vi "PWM.vi"(11 "Knob":dbl(knob) scale=0.0..100.0) -> (3 "s? t:f":bool)   [LabVIEW 2016]
panel:
  out "Waveform Chart":i16(graph)
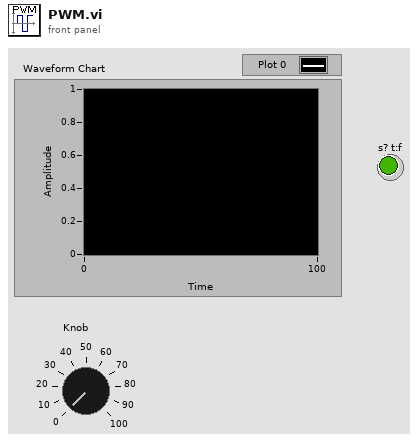
[diagram p1: front panel]
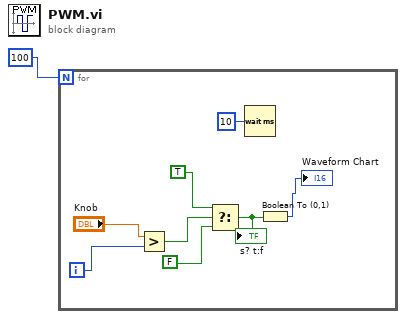
[diagram p0: block diagram]
diagram:
  n1 = for {
    N: 100 -> [_]
    i -> [w9]
    n2 = Greater?(x="Knob", y=w9) -> (0:w8:bool)
    n3 = Select(t=TRUE, s=w8, f=FALSE) -> (s? t:f=w4:bool)
    "s? t:f" <- w4
    n4 = Wait (ms)(milliseconds to wait=u32 10) -> ()  [unwired: 1 out]
    n5 = Boolean To (0,1)(Boolean=w4) -> (0, 1=→"Waveform Chart":i16)
  }
